vi "GET_PRODUCT_ID.vi"(11 "PRODFUCT_NAME":string="PRODUCT_NAME") -> (3 "PRODUCT_ID":string)   [LabVIEW 2020]
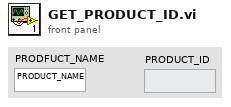
[diagram p1: front panel]
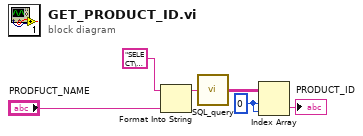
[diagram p0: block diagram]
diagram:
  w2 = 0 ("索引 (行)")
  n1 = Format Into String(format string="SELECT\ndbo.Product.PRODUCT_ID\n\nFROM\ndbo.Product\nWHERE\ndbo.Product.PRODUCT_NAME = '%s'\n" ("SQL query"), "PRODFUCT_NAME") -> (resulting string=w6:string)  [unwired: 2 in, 1 out]
  n2 = call "SQL_query.vi"("SQL query"=w6) -> ("data"=w3:string[][])  [unwired: 3 in, 1 out]
  n3 = Index Array(array=w3, index (row)=w2, index (col)=w2) -> (element=→"PRODUCT_ID":string)
